vi "Delete Custom Device VIs from Library (SubVI).vi"(8 "error out 2":errorcluster, 10 "Custom Device Library":path, 11 "Custom Device Project":path) -> (0 "error out":errorcluster)   [LabVIEW 2010]
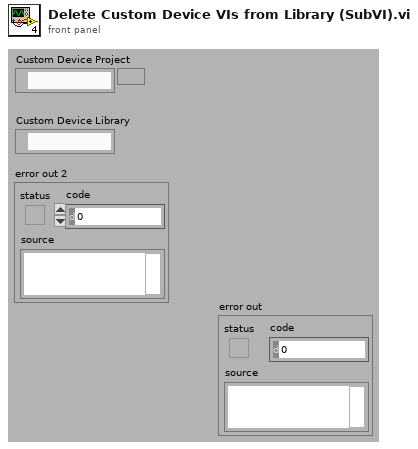
[diagram p1: front panel]
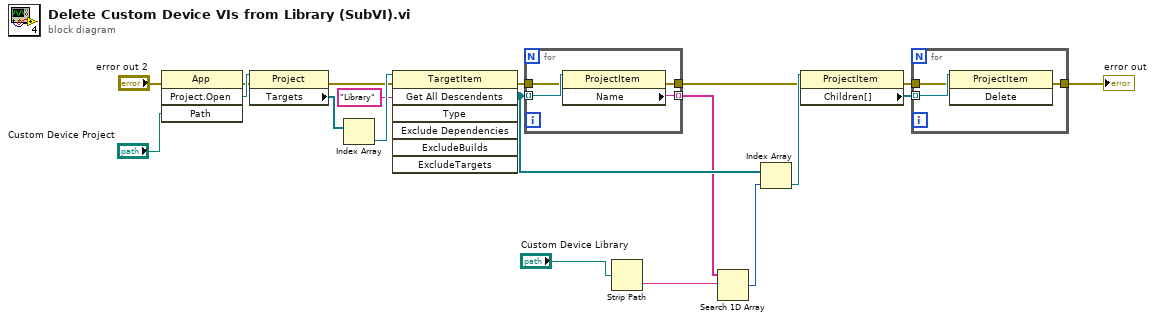
[diagram p0: block diagram]
diagram:
  n1 = invoke class="App" method="Project.Open"(error in="error out 2", "Path"="Custom Device Project") -> (error out=w3:errorcluster, "Project:Open"=w14:refnum<vi>)  [unwired: 2 in, 2 out]
  n2 = property class="Project"(reference=w14, error in=w3) -> (error out=w5:errorcluster, "Targets"=w4:refnum<vi>[])  [unwired: 1 out]
  n3 = Index Array(array=w4) -> (element=w13:refnum<vi>)  [unwired: 1 in]
  n4 = invoke class="TargetItem" method="Get All Descendents"(reference=w13, error in=w5, "Type"="Library") -> (error out=w9:errorcluster, "All Descendents"=w10:refnum<vi>[])  [unwired: 4 in, 5 out]
  n5 = for {
    tunnel: w10 -> [w23] mode=indexing
    tunnel: [w22] -> w8 mode=indexing
    tunnel: w9 -> [w21]
    tunnel: [w20] -> w11
    n6 = property class="ProjectItem"(reference=w23, error in=w21) -> (error out=w20:errorcluster, "Name"=w22:string)  [unwired: 1 out]
  }
  n7 = Strip Path(path="Custom Device Library") -> (name=w1:string)  [unwired: 1 out]
  n8 = Search 1D Array(1D array=w8, element=w1) -> (index of element=w12:i32)  [unwired: 1 in]
  n9 = Index Array(array=w10, index=w12) -> (element=w19:refnum<vi>)
  n10 = property class="ProjectItem"(reference=w19, error in=w11) -> (error out=w17:errorcluster, "Children[]"=w16:refnum<vi>[])  [unwired: 1 out]
  n11 = for {
    tunnel: w16 -> [w26] mode=indexing
    tunnel: w17 -> [w25]
    tunnel: [w24] -> w18
    n12 = invoke class="ProjectItem" method="Delete"(reference=w26, error in=w25) -> (error out=w24:errorcluster)  [unwired: 1 in, 2 out]
  }
  "error out" <- w18
